vi "current_t0.vi"() -> ()   [LabVIEW 2018]
panel:
  in  "t0 position":dbl
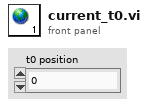
[diagram p1: front panel]
diagram:
